vi "Start.vi"(8 "Error In":errorcluster, 11 "object in":refnum<class "Rigol DS1054.lvclass">) -> (0 "Error Out":errorcluster, 3 "object out":refnum<class "Rigol DS1054.lvclass">)   [LabVIEW 2023, in "RIGOL DS1054.lvlib" / "Rigol DS1054.lvclass"]
uses:
  Rigol DS1054.lvclass
  Rigol DS1054.lvclass/Rigol DS1054.ctl
  <instrlib>/RIGOL DS1000 Series/RIGOL DS1000 Series.lvlib
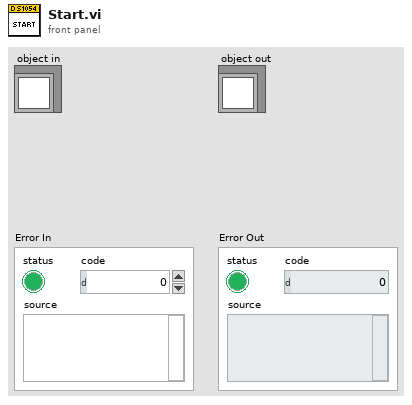
[diagram p1: front panel]
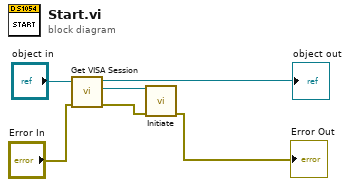
[diagram p0: block diagram]
diagram:
  n1 = call-dynamic "Get VISA Session.vi"("error in"="Error In", "Scope VISA in"="object in") -> ("error out"=w3:errorcluster, "VISA session"=w4:refnum<visa-resource-name>, "Scope VISA out"=→"object out":refnum<class "Rigol DS1054.lvclass">)  [unwired: 7 in]
  n2 = call <instrlib>:"Initiate.vi"("error in (no error)"=w3, "VISA resource name"=w4) -> ("error out"=→"Error Out":errorcluster)  [unwired: 8 in, 1 out]
